vi "StateQ.vi"(4 "QueueCommand":T3, 5 "error in (no error)":errorcluster, 8 "output cluster":T1) -> (0 "error out":errorcluster, 3 "queue out":refnum<queue>)   [LabVIEW 2018]
doc: "*-----------------------------------------------------\n* Author: SWatts\n*\n* VI Description: Sends Transitions to Wait for Transition\n* \n*\n* Error handling: All errors passed out\n*\n* Pre-condition: \n*\n* Post-condition: None\n*\n* Revision History:\n*\n* Rev Date Author Description \n* 01 30/04/2014 SWatts First issue\n*\n*-----------------------------------------------------"
uses:
  Controls/QueueCommand.ctl
  Controls/StateMessage.ctl
  Controls/Transition.ctl
panel:
  # "Input"
  # "Output"
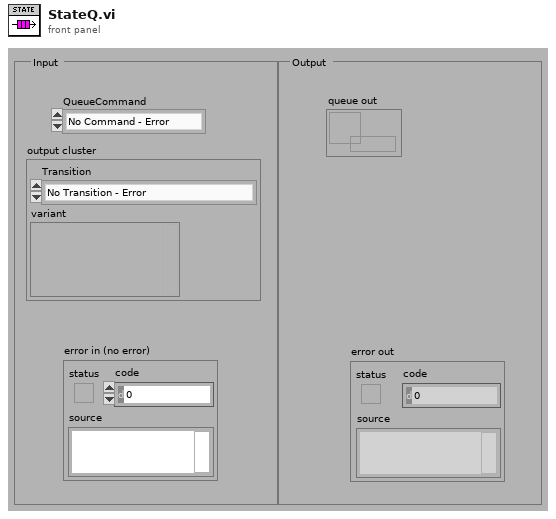
[diagram p1: front panel]
types:
  T1 = typedef "StateMessage.ctl" = cluster{"Transition":T2, "variant":variant}
  T2 = typedef "Transition.ctl" = enum16{"No Transition - Error", "Initialise", "Login", "Authenticate", "Log on Fail", "Login Success", "Logout", "Generate Error", "Start", "Stop", "Exit"}
  T3 = typedef "QueueCommand.ctl" = enum16{"No Command - Error", "Initialise", "Add to Bottom", "Add To Top", "Get Ref", "Close"}
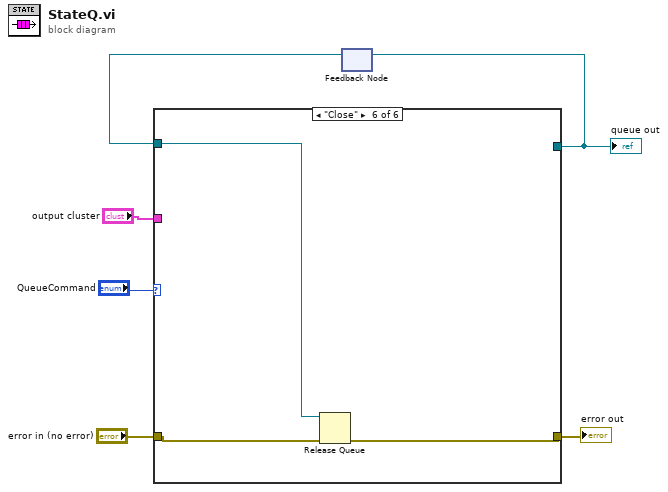
[diagram p0: block diagram]
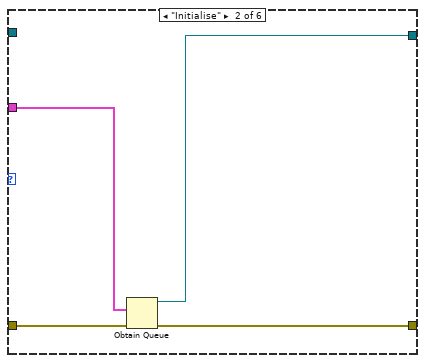
[diagram p3: hidden frame]
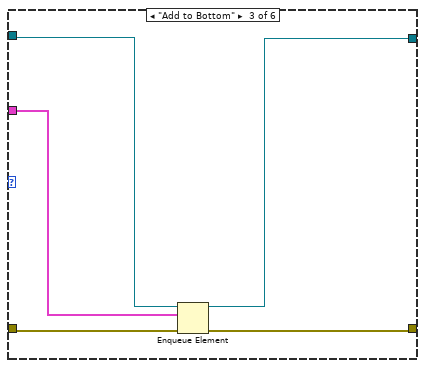
[diagram p4: hidden frame]
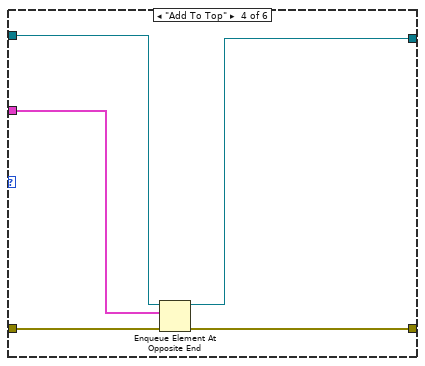
[diagram p5: hidden frame]
diagram:
  n1 = feedback #1() -> (w3:refnum<queue>)  [unwired: 1 in]
  n2 = case shown="\"Close\"" "QueueCommand" {
    tunnel: "output cluster" -> [_ w12 w13 w18 _ _]
    tunnel: [w8 w11 w14 w20 w24 _] -> w4
    tunnel: w3 -> [w8 _ w15 w19 w24 w25]
    tunnel: "error in (no error)" -> [w7 w10 w17 w22 w23 w27]
    tunnel: [w7 w9 w16 w21 w23 w26] -> w1
    frame "No Command - Error", Default {
    }
    frame "Initialise" {
      n3 = Obtain Queue(element data type=w12, error in (no error)=w10) -> (queue out=w11:refnum<queue>, error out=w9:errorcluster)  [unwired: 3 in, 1 out]
    }
    frame "Add to Bottom" {
      n4 = Enqueue Element(queue=w15, element=w13, error in (no error)=w17) -> (queue out=w14:refnum<queue>, error out=w16:errorcluster)  [unwired: 1 in, 1 out]
    }
    frame "Add To Top" {
      n5 = Enqueue Element At Opposite End(queue=w19, element=w18, error in (no error)=w22) -> (queue out=w20:refnum<queue>, error out=w21:errorcluster)  [unwired: 1 in, 1 out]
    }
    frame "Get Ref" {
    }
    frame "Close" {
      n6 = Release Queue(queue=w25, error in (no error)=w27) -> (error out=w26:errorcluster)  [unwired: 1 in, 2 out]
    }
  }
  "error out" <- w1
  "queue out" <- w4
  n7 = feedback-in #1(w4) -> ()
